vi "FlashLEDs.vi"(7 "LED line":tag, 8 "error in (no error)":errorcluster, 10 "LED off (s)":dbl, 11 "LED on (s)":dbl) -> (0 "error out":errorcluster)   [LabVIEW 2017, in "Scope.lvlib" / "Trigger.lvlib"]
uses:
  Trigger.lvlib
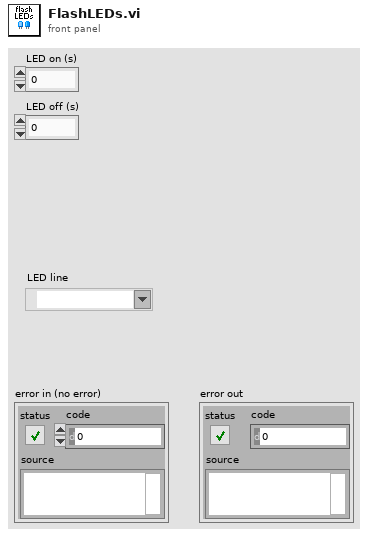
[diagram p1: front panel]
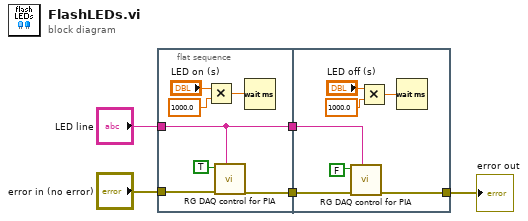
[diagram p0: block diagram]
diagram:
  n1 = flat-sequence {
    tunnel: [w10] -> w2
    tunnel: [w6] -> w1
    tunnel: "error in (no error)" -> [w11]
    tunnel: "LED line" -> [w6]
    tunnel: [w16] -> w4
    tunnel: w2 -> [w17]
    tunnel: w1 -> [w13]
    frame #0 {
      n2 = Multiply(x="LED on (s)", y=1000.0) -> (x*y=w7:dbl)
      n3 = call "RG DAQ control for PIA.vi"("LED line"=w6, "error in"=w11, "value"=TRUE ("Initial value")) -> ("error out"=w10:errorcluster)  [unwired: 8 in]
      n4 = Wait (ms)(milliseconds to wait=w7) -> ()  [unwired: 1 out]
    }
    frame #1 {
      n5 = call "RG DAQ control for PIA.vi"("LED line"=w13, "error in"=w17, "value"=FALSE ("Initial value")) -> ("error out"=w16:errorcluster)  [unwired: 8 in]
      n6 = Multiply(x="LED off (s)", y=1000.0) -> (x*y=w15:dbl)
      n7 = Wait (ms)(milliseconds to wait=w15) -> ()  [unwired: 1 out]
    }
  }
  "error out" <- w4
